vi "Exemple_Extraction_Reconstruct_From_Patches_2D.vi"() -> ()   [LabVIEW 2020]
uses:
  Objet/6 - Datasets Transformation/6.2 - Feature extraction/PatchExtractor/PatchExtractor.lvclass
panel:
  out "Data":T1
  in  "Image":u16(ring) items=["China", "Flower"]
  in  "PatchExtractor":T2={"patch_size"={"patch_height"=2, "patch_width"=2}, "max_patches"="None", "random_state"=-1} {"random_state" min=-1}
  out "error out":errorcluster caption="sortie d'erreur"
  in  "error in":errorcluster caption="entrée d'erreur"
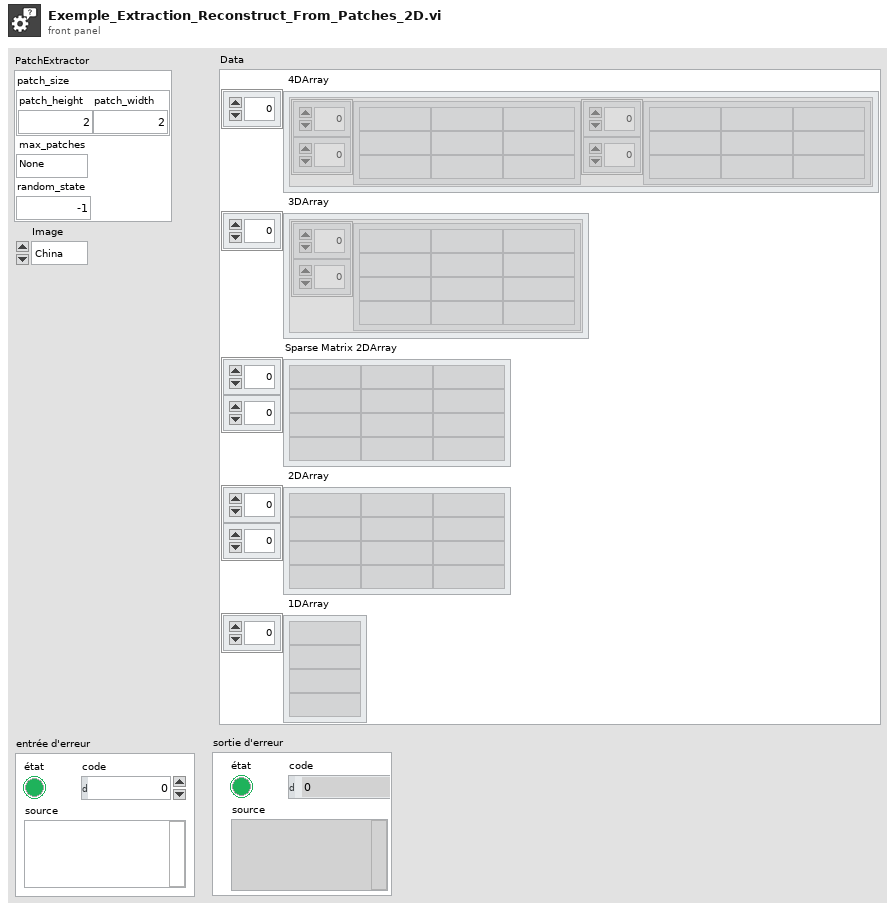
[diagram p1: front panel]
types:
  T1 = cluster{" 4DArray":cluster{"1":string[][], "2":string[][]}[], " 3DArray":cluster{"Tableau":string[][]}[], "Sparse Matrix 2DArray":string[][], " 2DArray":string[][], " 1DArray":string[]}
  T2 = cluster{"patch_size":cluster{"patch_height":i32, "patch_width":i32}, "max_patches":string, "random_state":i32}
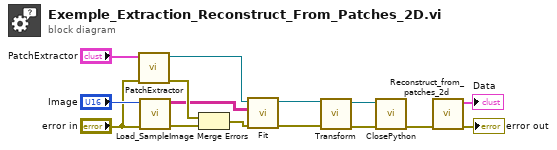
[diagram p0: block diagram]
diagram:
  n1 = call "PatchExtractor.vi"("error in"="error in", "PatchExtractor"="PatchExtractor") -> ("error out"=w7:errorcluster, "PatchExtractor.lvclass"=w10:refnum<class "PatchExtractor.lvclass">)  [unwired: 8 in]
  n2 = call "Load_SampleImage.vi"("error in"="error in", "Image"="Image") -> ("error out"=w11:errorcluster, "Image (RGB)"=w5:string[][])  [unwired: 8 in]
  n3 = Merge Errors(w7, w11) -> (w8:errorcluster)
  n4 = call-dynamic "Fit.vi"("error in (no error)"=w8, "Image"=w5, "PatchExtractor.lvclass"=w10) -> ("error out"=w12:errorcluster, "PatchExtractor.lvclass"=w9:refnum<class "PatchExtractor.lvclass">)  [unwired: 6 in, 1 out]
  n5 = call-dynamic "Transform.vi"("error in (no error)"=w12, "PatchExtractor.lvclass"=w9) -> ("error out"=w2:errorcluster, "PatchExtractor.lvclass"=w3:refnum<class "PatchExtractor.lvclass">)  [unwired: 7 in, 1 out]
  n6 = call-dynamic "ClosePython.vi"("error in (no error)"=w2, "Scikit-learn en entrée"=w3) -> ("error out"=w1:errorcluster)  [unwired: 8 in, 1 out]
  n7 = call "Reconstruct_from_patches_2d.vi"("error in"=w1) -> ("error out"=→"error out":errorcluster, "Data"=→"Data":T1)  [unwired: 9 in]
